vi "CS_cRIO-PB_DP-Slave_GetSetAddress.vi"(0 "FPGA VI Reference":T1, 2 "Mode":enum16{"Get", "Set"}(ring), 7 "Set address":u8, 11 "Error":errorcluster) -> (4 "FPGA VI Reference out":T1, 8 "Get address":u8, 15 "Error out":errorcluster)   [LabVIEW 2013, in "dynamic profibus.lvlib"]
doc: "Handles the cyclic process data of the selected DP-Slave.\n\nFPGA VI Reference:\nReference of the FPGA VI.\n\nSlave:\nPROFIBUS address of the DP-Slave. \n\nModify output data:\nThe Modify output data array contains the DP-Slave output data to be changed.\n\nInput data:\nThe Input data array contains the DP-Slave input data.\n\nOutput data:\nThe Output data array contains the DP-Slave output data.\n\nInput length:\nReturns the configured input length of the DP-Slave.\n\nOutput length:\nReturns the configured output length of the DP-Slave.\n\nSlave status:\n0x00: DP-Slave is in DataExchange mode, input and output data are valid\n0xC3: DP-Slave is not in Data Exchange mode, input and output data are invalid, DP-Slave diagnostic data are reported in Diag data array\n0xFF: DP-Slave is in Data Exchange mode and reports ext. diagnostic data, input and output data are valid.\n\nFPGA VI Reference out:\nIs a copy of the FPGA VI Reference .\n\nError in:\nPreceding error conditions. If an error has already occurred, the VI returns the value of the error in Error out.\n\nError out:\nError: TRUE if an error occurred.\nStatus: Error code\nInfo: Error description"
uses:
  dynamic profibus.lvlib
  CS_cRIO-PB_DP-Slave_FPGA-Reference.ctl
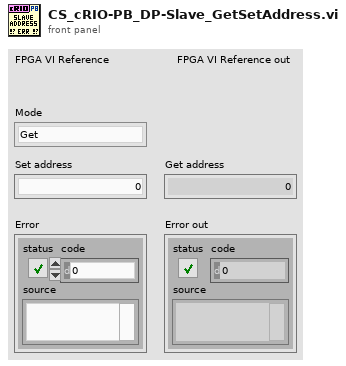
[diagram p1: front panel]
types:
  T1 = typedef "dynamic profibus.lvlib/CS_cRIO-PB_DP-Slave_FPGA-Reference.ctl" = refnum<k20>
  T2 = enum16{"Get DP-AutoSlave Address", "Set DP-AutoSlave Address", "Get Slave Output Data", "Set Slave Input Data", "Read/Write Slave Data"}
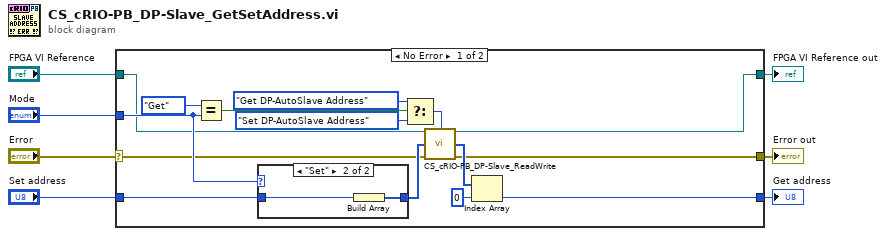
[diagram p0: block diagram]
diagram:
  n1 = case shown="No Error" "Error" {
    selector: "Error" -> [w18 w25]
    tunnel: "FPGA VI Reference" -> [w21 w26]
    tunnel: [w17 w26] -> w5
    tunnel: [w16 w25] -> w4
    tunnel: "Mode" -> [w22 _]
    tunnel: "Set address" -> [w15 _]
    tunnel: [w14 _] -> w1
    frame No Error {
      n2 = Equal?(x=enum16{"Get", "Set"}."Get", y=w22) -> (x = y?=w12:bool)
      n3 = case shown="\"Set\"" w22 {
        tunnel: w15 -> [_ w24]
        tunnel: [_ w23] -> w19
        frame "Get" {
        }
        frame "Set" {
          n4 = Build Array(w24) -> (w23:u8[])
        }
      }
      n5 = Select(t=T2."Get DP-AutoSlave Address" ("Mode"), s=w12, f=T2."Set DP-AutoSlave Address" ("Mode")) -> (s? t:f=w8:T2)
      n6 = call "CS_cRIO-PB_DP-Slave_ReadWrite.vi"("FPGA VI Reference"=w21, "Mode"=w8, "Data"=w19, "Error"=w18) -> ("FPGA VI Reference out"=w17:T1, "Data out"=w20:u8[], "Error out"=w16:errorcluster)  [unwired: 8 in, 1 out]
      n7 = Index Array(array=w20, index=0) -> (element=w14:u8)
    }
    frame Error {
    }
  }
  "FPGA VI Reference out" <- w5
  "Error out" <- w4
  "Get address" <- w1
